vi "PWM_General_v1.vi"(7 "ControlBoard VISA":refnum<visa-resource-name>, 8 "error in (no error)":errorcluster, 9 "Limits":T2={"Expected Duty Cycle"=25, "Duty Cycle Error"=1.0, "Expected Frequency"=2500.0, "Frequency Error"=0.5, "Expected Vrms"=15.8, "Vrms Error"=5.0, "Expected Vdc HIGH"=0.5, "Expected Vdc LOW"=-0.5, "Expected Vrms HIGH"=1.0} {"Expected Vrms HIGH" format="%#_13g"; "Expected Vdc LOW" format="%#_13g"; "Expected Vdc HIGH" format="%#_13g"; "Expected Vrms" format="%#_13g"; "Expected Frequency" format="%#_13g"}, 10 "Legs (3 or 6)":enum16{"3 Legs", "6 Legs"}(ring), 11 "Task Select":T1(ring)) -> (0 "error out":errorcluster, 1 "data":waveform(dbl)[](array[waveform]), 2 "Message OUT":string, 3 "Result":bool)   [LabVIEW 2022 SP3]
doc: "This VI will cause each leg to gate, and will output the results."
uses:
  <vilib>/DAQmx/read.llb/DAQmx Read (Analog 1D Wfm NChan NSamp).vi
  <vilib>/DAQmx/miscellaneous.llb/DAQmx Fill In Error Info.vi
panel:
  in  "Message IN":string=" "
  out "Analysis Leg":i32
  out "Waveforms":T3
  out "Active Leg":i32
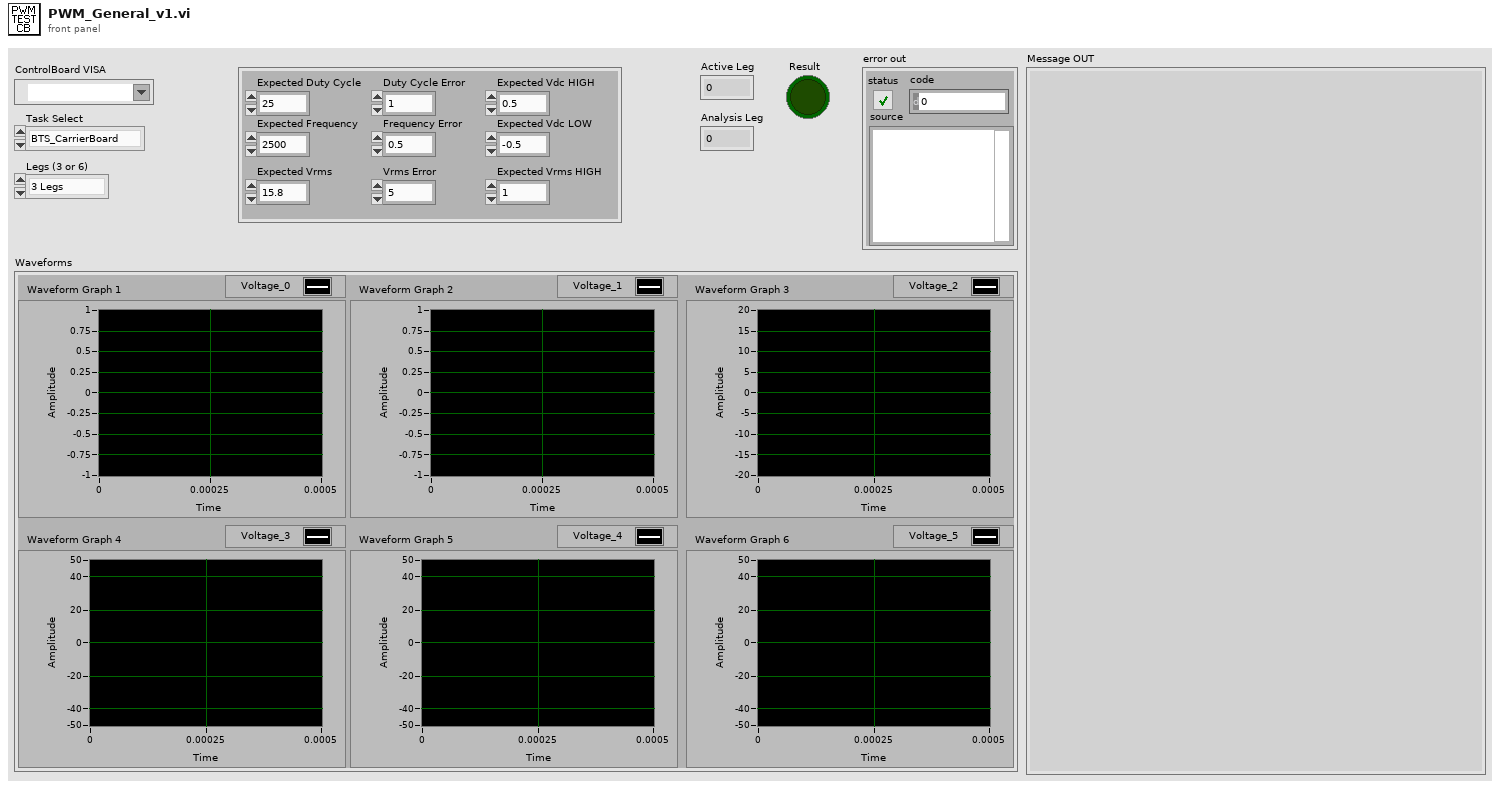
[diagram p1: front panel]
types:
  T1 = enum16{"BTS_CarrierBoard", "BTS_ControlBoard", "FTS2_3Outputs", "FTS2_6Outputs"}
  T2 = cluster{"Expected Duty Cycle":i32, "Duty Cycle Error":dbl, "Expected Frequency":dbl, "Frequency Error":dbl, "Expected Vrms":dbl, "Vrms Error":dbl, "Expected Vdc HIGH":dbl, "Expected Vdc LOW":dbl, "Expected Vrms HIGH":dbl}
  T3 = cluster{"Waveform Graph 1":waveform(dbl), "Waveform Graph 2":waveform(dbl), "Waveform Graph 3":waveform(dbl), "Waveform Graph 4":waveform(dbl), "Waveform Graph 5":waveform(dbl), "Waveform Graph 6":waveform(dbl)}
  T4 = cluster{"data[0]":waveform(dbl), "data[1]":waveform(dbl), "data[2]":waveform(dbl), "data[3]":waveform(dbl), "data[4]":waveform(dbl), "data[5]":waveform(dbl)}
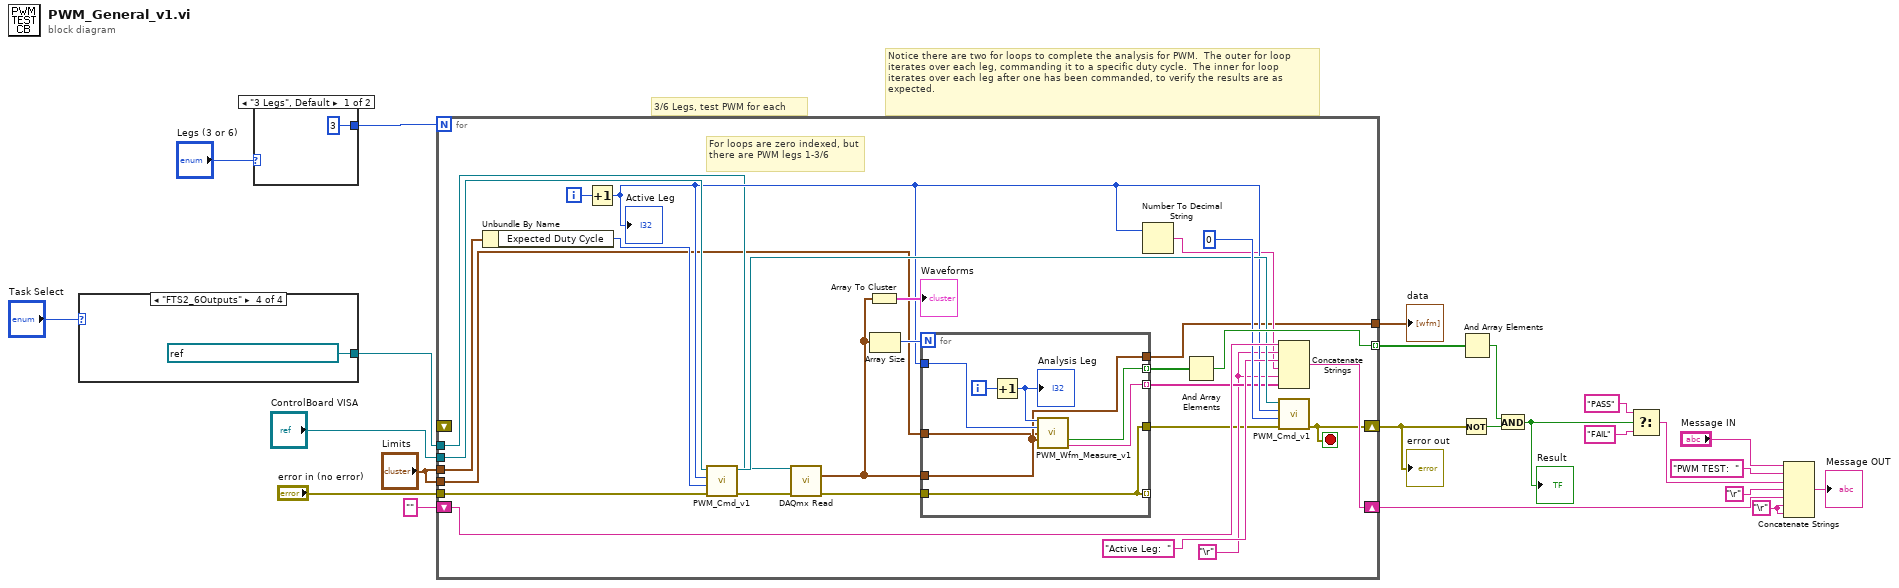
[diagram p0: block diagram]
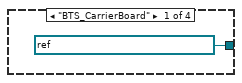
[diagram p2: hidden frame]
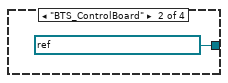
[diagram p3: hidden frame]
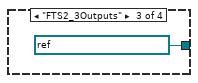
[diagram p4: hidden frame]
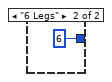
[diagram p5: hidden frame]
diagram:
  w17 = "\r"
  # "Notice there are two for loops to complete the analysis for PWM.  The outer for loop iterates over each leg, commanding it to a specific duty cycle.  The inner for loop iterates over each leg after one has been commanded, to verify the results are as expected."
  # "3/6 Legs, test PWM for each"
  n1 = case shown="\"FTS2_6Outputs\"" "Task Select" {
    tunnel: [refnum<k21> "BTS_PWMInput_CarrierBoard" ("task/channels in") refnum<k21> "BTS_PWMInput_Hydra_CB" ("task/channels in") refnum<k21> "FTS2_PWMInput_DG" ("task/channels in") refnum<k21> "FTS2_PWMInput_Hydra_CB" ("task/channels in")] -> w6
    frame "BTS_CarrierBoard" {
    }
    frame "BTS_ControlBoard" {
    }
    frame "FTS2_3Outputs" {
    }
    frame "FTS2_6Outputs" {
    }
  }
  n2 = case shown="\"3 Legs\", Default" "Legs (3 or 6)" {
    tunnel: [3 6] -> w4
    frame "3 Legs", Default {
    }
    frame "6 Legs" {
    }
  }
  n3 = for {
    N: w4 -> [_]
    tunnel: "ControlBoard VISA" -> [w50]
    tunnel: [w55] -> w23 mode=indexing
    shift-right: [w54] -> w15
    shift-left: "" -> [w53]
    shift-right: [w37] -> w9
    shift-left: _ -> [_]
    tunnel: "error in (no error)" -> [w35]
    tunnel: w6 -> [w34]
    tunnel: [w33] -> w3
    tunnel: "Limits" -> [w31]
    tunnel: "Limits" -> [w30]
    i -> [w49]
    stop <- w37 stop-if-true
    w40 = "\r"
    # "For loops are zero indexed, but there are PWM legs 1-3/6"
    n4 = Unbundle By Name(w30) -> ("Expected Duty Cycle"=w32:i32)
    n5 = Increment(x=w49) -> (x+1=w42:i32)
    "Active Leg" <- w42
    n6 = call "PWM_Cmd_v1.vi"("error in (no error)"=w35, "Duty Cycle"=w32, "Leg"=w42, "VISA Refnum in"=w50) -> ("error out"=w44:errorcluster, "VISA Refnum out"=w51:refnum<visa-resource-name>)  [unwired: 5 in, 1 out]
    n7 = call-poly <vilib>:"DAQmx Read.vi"("task/channels in"=w34, "error in"=w44) -> ("data"=w45:waveform(dbl)[], "error out"=w38:errorcluster)  [unwired: 11 in, 1 out]
    n8 = Array To Cluster(array=w45) -> (cluster=→"Waveforms":T4)
    n9 = Array Size(array=w45) -> (size(s)=w46:i32)
    n10 = for {
      N: w46 -> [_]
      tunnel: w45 -> [w57]
      tunnel: w42 -> [w63]
      tunnel: [w60] -> w47 mode=indexing
      tunnel: [w59] -> w41 mode=indexing
      tunnel: w38 -> [w58]
      tunnel: [w58] -> _ mode=indexing
      tunnel: [w58] -> w36
      tunnel: [w57] -> w33
      tunnel: w31 -> [w56]
      i -> [w62]
      n11 = Increment(x=w62) -> (x+1=w61:i32)
      "Analysis Leg" <- w61
      n12 = call "PWM_Wfm_Measure_v1.vi"("Analysis Leg"=w61, "Active Leg"=w63, "Limits"=w56, "Waveform"=w57) -> ("Result (Boolean)"=w60:bool, "Message"=w59:string)  [unwired: 9 in, 1 out]
    }
    n13 = Number To Decimal String(number=w42) -> (decimal integer string=w39:string)  [unwired: 1 in]
    n14 = And Array Elements(Boolean array=w47) -> (logical AND=w55:bool)
    n15 = Concatenate Strings(w53, w40, "Active Leg:  ", w39, w40, w41) -> (w54:string)
    n16 = call "PWM_Cmd_v1.vi"("error in (no error)"=w36, "Duty Cycle"=0, "Leg"=w42, "VISA Refnum in"=w51) -> ("error out"=w37:errorcluster)  [unwired: 5 in, 2 out]
  }
  "error out" <- w9
  "data" <- w3
  n17 = Not(x=w9) -> (.not. x?=w20:bool)
  n18 = And Array Elements(Boolean array=w23) -> (logical AND=w18:bool)
  n19 = And(x=w18, y=w20) -> (x .and. y?=w19:bool)
  "Result" <- w19
  n20 = Select(t="PASS", s=w19, f="FAIL") -> (s? t:f=w10:string)
  n21 = Concatenate Strings("Message IN", "PWM TEST:  ", w10, "\r", w15, w17, w17) -> (→"Message OUT":string)
